vi "B4_Create.vi"(8 "error in (no error)":errorcluster, 11 "reference in":refnum<class "B4.lvclass">) -> (0 "error out":errorcluster, 3 "reference out":refnum<class "B4.lvclass">)   [LabVIEW 2012, in "B4.lvclass"]
uses:
  B4.lvclass
  A4_class/A4.lvclass
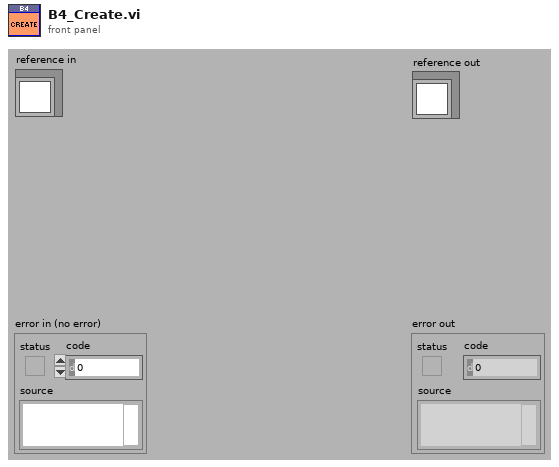
[diagram p1: front panel]
types:
  T1 = typedef "G4SubTemplate_Simple_4x4x4.lvclass/ObjectAttributes.ctl" = cluster{"Attribute1":dbl}
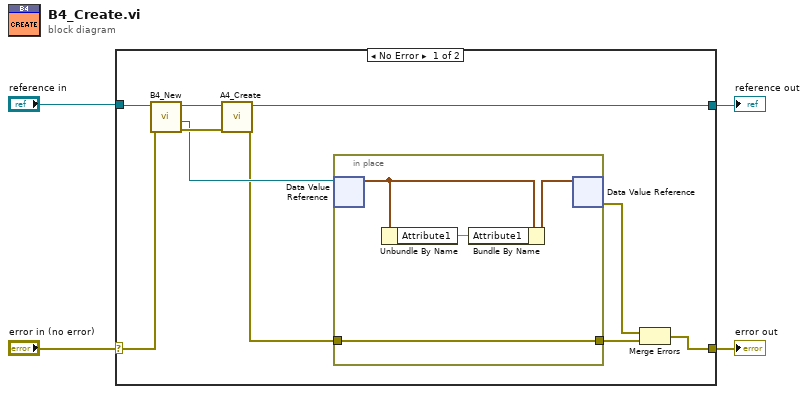
[diagram p0: block diagram]
diagram:
  n1 = case shown="No Error" "error in (no error)" {
    selector: "error in (no error)" -> [w11 w20]
    tunnel: [w9 w20] -> w3
    tunnel: "reference in" -> [w13 w19]
    tunnel: [w8 w19] -> w1
    frame No Error {
      n2 = call "B4_New.vi"("error in (no error)"=w11, "reference in"=w13) -> ("error out"=w12:errorcluster, "DVRRefOut"=w7:refnum<data-value>, "reference out"=w14:refnum<class "B4.lvclass">)  [unwired: 6 in, 1 out]
      n3 = call "A4_Create.vi"("error in (no error)"=w12, "reference in"=w14) -> ("error out"=w6:errorcluster, "reference out"=w8:refnum<class "B4.lvclass">)  [unwired: 8 in]
      n4 = in-place {
        in-place-border: w6 -> [w15]
        in-place-border: [w15] -> w5
        n5 = in-place-dvr #1(w7) -> (w17:T1)  [unwired: 1 out]
        n6 = Unbundle By Name(w17) -> ("Attribute1"=w16:dbl)
        n7 = Bundle By Name(cluster=w17, "Attribute1"=w16) -> (w18:T1)
        n8 = in-place-dvr #1(w18) -> (w10:errorcluster)  [unwired: 1 out]
      }
      n9 = Merge Errors(w10, w5) -> (w9:errorcluster)
    }
    frame Error {
    }
  }
  "error out" <- w3
  "reference out" <- w1
